vi "Fetch All Segments.vi"(4 "Sparsing (0: Every point)":i16, 5 "Number of points (0: All points)":i16, 7 "First point (0: First point)":i16, 8 "error in (no error)":errorcluster, 9 "Timeout (10000 ms)":u32=10000, 10 "Source (0: Channel 1)":u16(ring) items=["Channel 1", "Channel 2", "Channel 3", "Channel 4", "Memory 1", "Memory 2", "Memory 3", "Memory 4", "Function 1", "Function 2", "Function 3", "Function 4", "Function 5", "Function 6", "Function 7", "Function 8"], 11 "VISA resource name":refnum<visa-resource-name>) -> (0 "error out":errorcluster, 2 "Array":waveform(dbl)[](array[waveform]), 3 "VISA resource name out":refnum<visa-resource-name>)   [LabVIEW 2020, in "LeCroy Wave Series.lvlib"]
doc: "Returns the alls segments of waveform the oscilloscope acquired for the specified channel. The waveform is from an acquisition that you initiate prior to calling this VI.\n\nYou use the Initiate VI to start an acquisition on the channels that you enable with the <B>Configure Channel</B> VI. The oscilloscope acquires waveforms for the enabled channels concurrently. You must call this VI separately for each enabled channel to obtain the waveforms.\n\nYou can call the <B>lcwave Read Single Segment</B> VI or <B>lcwave Read Multiple Segments</B> VI instead of using low level VIs.\n\n<B>Note</B> This VI does not check the instrument status. Typically, you call this VI only in a sequence of calls to other low-level instrument driver VIs. The sequence performs one operation. You use the low-level VIs to optimize one or more aspects of interaction with the instrument."
uses:
  LeCroy Wave Series.lvlib
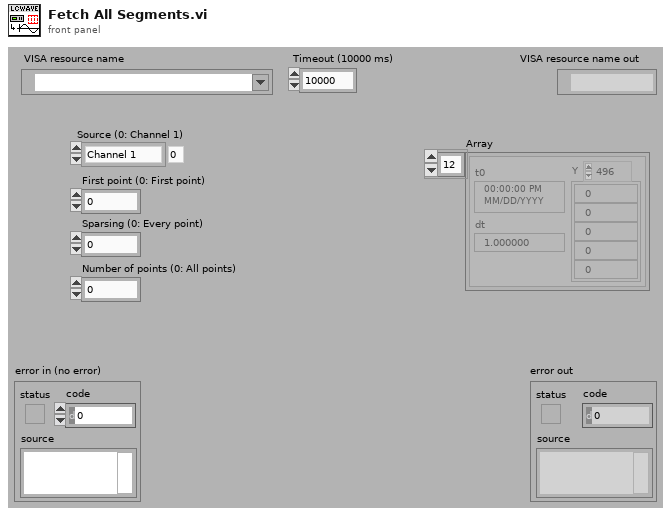
[diagram p1: front panel]
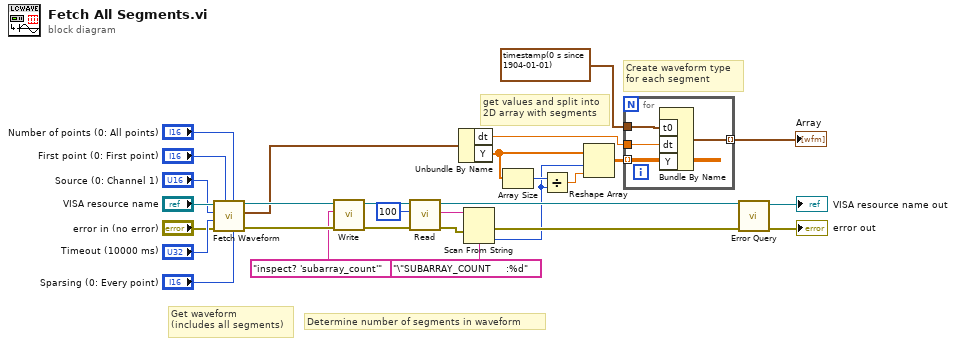
[diagram p0: block diagram]
diagram:
  # "Create waveform type\nfor each segment"
  # "get values and split into\n2D array with segments"
  # "Determine number of segments in waveform"
  # "Get waveform\n(includes all segments)"
  n1 = call "Fetch Waveform.vi"("Sparsing (0: Every point)"="Sparsing (0: Every point)", "Number of points (0: All points)"="Number of points (0: All points)", "First point (0: First point)"="First point (0: First point)", "error in (no error)"="error in (no error)", "Timeout (10000 ms)"="Timeout (10000 ms)", "Source (0: Channel 1)"="Source (0: Channel 1)", "VISA resource name"="VISA resource name") -> ("error out"=w20:errorcluster, "Waveform Graph"=w8:waveform(dbl), "VISA resource name out"=w19:refnum<visa-resource-name>)  [unwired: 2 in]
  n2 = call "Write.vi"("error in (no error)"=w20, "Write Buffer"="inspect? 'subarray_count'", "VISA resource name"=w19) -> ("error out"=w17:errorcluster, "VISA resource name out"=w21:refnum<visa-resource-name>)  [unwired: 6 in, 1 out]
  n3 = call "Read.vi"("error in (no error)"=w17, "Byte Count"=u32 100, "VISA resource name"=w21) -> ("error out"=w13:errorcluster, "Read Buffer"=w15:string, "VISA resource name out"=w5:refnum<visa-resource-name>)  [unwired: 5 in, 1 out]
  n4 = Unbundle By Name(w8) -> ("dt"=w3:dbl, "Y"=w11:dbl[])
  n5 = Scan From String(format string="\"SUBARRAY_COUNT     :%d", input string=w15, error in=w13) -> (error out=w4:errorcluster, output 1=w2:i32)  [unwired: 2 in, 2 out]
  n6 = Array Size(array=w11) -> (size(s)=w10:i32)
  n7 = Divide(x=w10, y=w2) -> (x/y=w9:dbl)
  n8 = Reshape Array(w11, w2, w9) -> (w7:dbl[][])
  n9 = for {
    tunnel: w7 -> [w33] mode=indexing
    tunnel: w3 -> [w32]
    tunnel: [w31] -> w6 mode=indexing
    tunnel: timestamp(0 s since 1904-01-01) ("t0") -> [w30]
    n10 = Bundle By Name("t0"=w30, "dt"=w32, "Y"=w33) -> (w31:waveform(dbl))  [unwired: 1 in]
  }
  "Array" <- w6
  n11 = call "Error Query.vi"("error in (no error)"=w4, "VISA resource name"=w5) -> ("error out"=→"error out":errorcluster, "VISA resource name out"=→"VISA resource name out":refnum<visa-resource-name>)  [unwired: 6 in, 2 out]
